vi "Averaged FFT Spectrum (Real-Im).vi"(0 "scaled signal [EU]":dbl[](array[numeric]) format="%.2f", 1 "sampling frequency [Hz]":dbl=10000.0 format="%.2f", 2 "window":T6 items=["Rectangle"=0, "Hanning"=1, "Hamming"=2, "Blackman-Harris"=3, "Exact Blackman"=4, "Blackman"=5, "Flat Top"=6, "4 Term B-Harris "=7, "7 Term B-Harris"=8, "Low Sidelobe"=9, "Blackman Nuttall"=11, "Triangle"=30, "Bartlett-Hanning"=31, "Bohman"=32, "Parzen"=33, "Welch"=34, "Kaiser"=60, "Dolph-Chebyshev"=61, "Gaussian"=62], 5 "channel info":T1={"sensor sensitivity [mV/EU]"=1000.0, "engineering units"=1, "dB reference [EU]"=1.0, "custom label"="EU", "weighting filter"=0, "pregain [dB]"=0.0} {"pregain [dB]" format="%.2f"; "weighting filter" items=["Linear", "A-weighting", "B-weighting", "C-weighting", "ITU-R 468-4", "Dolby", "CCITT", "C-message"]; "dB reference [EU]" format="%^.1e"; "engineering units" items=["custom..."=0, "V"=1, "A"=21, "Pa"=2, "N"=20, "g"=3, "m/s^2"=4, "m/s"=5, "m"=6, "mm/s"=12, "mm"=13, "microns/s"=14, "microns"=15, "in/s^2"=7, "in/s"=8, "in"=9, "mils/s"=10, "mils"=11, "rad/s^2"=16, "rad/s"=17, "rad"=18, "strain"=19]; "sensor sensitivity [mV/EU]" format="%.2f"}, 6 "frequency weighting":T5(ring), 7 "reset averaging (T)":bool=TRUE, 9 "averaging parameters":T4={"averaging mode"=enum."RMS averaging", "weighting mode"=enum."Linear", "number of averages"=10} {"number of averages" min=1}) -> (11 "window constants":cluster{"eq noise BW":dbl, "coherent gain":dbl} {"coherent gain" format="%.2f"; "eq noise BW" format="%.2f"}, 12 "df [Hz]":dbl format="%.2f", 13 "weighting conflict":bool, 14 "real part [EUrms]":dbl[](array[numeric]) format="%.2f", 15 "imaginary part [EUrms]":dbl[](array[numeric]) format="%.2f", 16 "unit label":string, 18 "averages completed":dbl format="%.2f", 19 "error out":errorcluster)   [LabVIEW 2017]
doc: "Computes the averaged FFT spectrum of the input signal. FFT results are returned as real and imaginary parts.\nEach block of data corresponds to a single FFT block and has to be passed individually to this VI. The first time this VI is called, reset averaging must be TRUE (default value), to start a new averaging process. For subsequent calls, reset averaging must be FALSE to continue the averaging process. Averages completed returns the number of averages completed so far.\nAveraging parameters specifies how the averaging is performed. This includes the averaging mode (no averaging, vector averaging, RMS averaging, or peak hold), the weighting mode (linear or exponential), and the number of averages (used only if the weighting mode is exponential).\nThe selected frequency weighting (A, B, or C) is applied to the results in the frequency domain. There is no time-domain filtering operation."
uses:
  <vilib>/Analysis/4window.llb/windowTd.ctl
  <vilib>/addons/Sound and Vibration/compatibility/Controls/svl_Channel Info.ctl
  <vilib>/addons/Sound and Vibration/compatibility/Controls/svl_Engineering Units Text Ring.ctl
  <vilib>/addons/Sound and Vibration/compatibility/Controls/svl_Weighting Filter Text Ring.ctl
  <vilib>/Analysis/2dsp.llb/Real FFT.vi
  <vilib>/Analysis/2dsp.llb/Power Spectrum (DBL).vi
  <vilib>/Analysis/0measdsp.llb/Scaled Time Domain Window (DBL).vi
  <vilib>/Analysis/NI_AALPro.lvlib
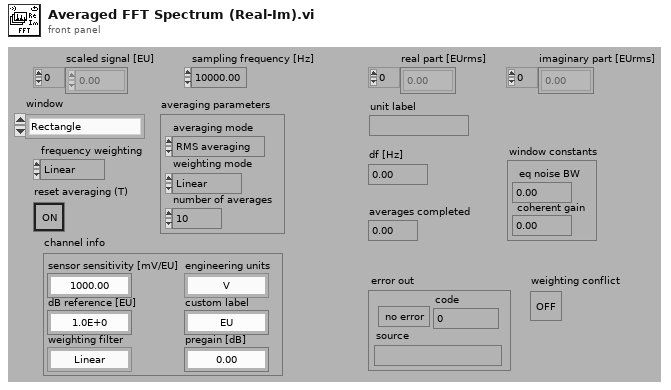
[diagram p1: front panel]
types:
  T1 = typedef "svl_Channel Info.ctl" = cluster{"sensor sensitivity [mV/EU]":dbl, "engineering units":T2, "dB reference [EU]":dbl, "custom label":string, "weighting filter":T3, "pregain [dB]":dbl}
  T2 = typedef "svl_Engineering Units Text Ring.ctl" = u16
  T3 = typedef "svl_Weighting Filter Text Ring.ctl" = u16
  T4 = cluster{"averaging mode":enum16{"No averaging", "Vector averaging", "RMS averaging", "Peak hold"}, "weighting mode":enum16{"Linear", "Exponential"}, "number of averages":u32}
  T5 = enum16{"Linear", "A-weighting", "B-weighting", "C-weighting"}
  T6 = typedef "NI_AALPro.lvlib/windowTd.ctl" = u32
  T7 = enum16{"No averaging", "Vector averaging", "RMS averaging", "Peak hold"}
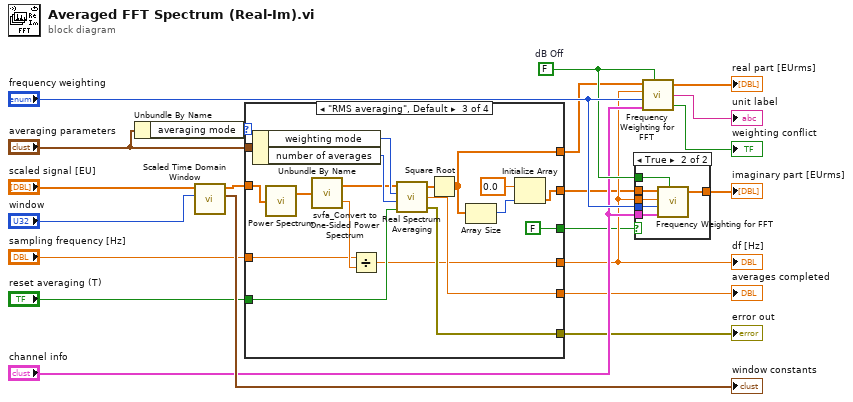
[diagram p0: block diagram]
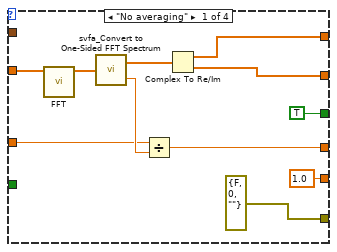
[diagram p2: hidden frame]
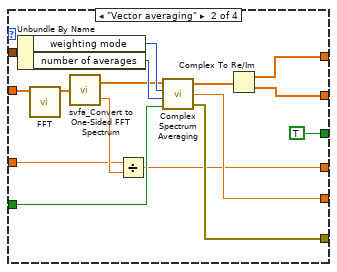
[diagram p3: hidden frame]
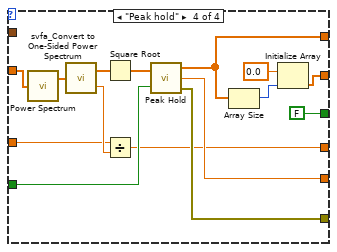
[diagram p4: hidden frame]
diagram:
  w17 = FALSE  # dB Off
  n1 = Unbundle By Name("averaging parameters") -> ("averaging mode"=w8:T7)
  n2 = call-poly <vilib>:"Scaled Time Domain Window.vi"("window"="window", "X"="scaled signal [EU]") -> ("window properties"=→"window constants":cluster{"eq noise BW":dbl, "coherent gain":dbl}, "Windowed X"=w10:dbl[])  [unwired: 7 in, 1 out]
  n3 = case shown="\"RMS averaging\", Default" w8 {
    tunnel: "sampling frequency [Hz]" -> [w23 w34 w50 w69]
    tunnel: [w22 w33 w49 w68] -> w6
    tunnel: [1.0 ("averages completed") w48 w65 w79] -> w7
    tunnel: "reset averaging (T)" -> [_ w47 w66 w80]
    tunnel: w10 -> [w25 w36 w52 w70]
    tunnel: "averaging parameters" -> [_ w46 w64 _]
    tunnel: [w31 w44 w56 w75] -> w3
    tunnel: [w30 w43 w63 w76] -> w4
    tunnel: [TRUE TRUE FALSE FALSE] -> w5
    tunnel: [errorcluster {"status"=FALSE, "code"=0, "source"=""} ("error out") w39 w59 w73] -> w2
    frame "No averaging" {
      n4 = call-poly <vilib>:"FFT.vi"("X"=w25) -> ("FFT {X}"=w27:cdb[])  [unwired: 9 in, 1 out]
      n5 = call <vilib>:"svfa_Convert to One-Sided FFT Spectrum.vi"("two-sided FFT spectrum"=w27) -> ("one-sided FFT spectrum"=w24:cdb[], "block size"=w26:dbl)
      n6 = Divide(x=w23, y=w26) -> (x/y=w22:dbl)
      n7 = Complex To Re/Im(x + iy=w24) -> (x=w31:dbl[], y=w30:dbl[])
    }
    frame "Vector averaging" {
      n8 = Unbundle By Name(w46) -> ("weighting mode"=w41:enum16{"Linear", "Exponential"}, "number of averages"=w40:u32)
      n9 = call-poly <vilib>:"FFT.vi"("X"=w36) -> ("FFT {X}"=w38:cdb[])  [unwired: 9 in, 1 out]
      n10 = call <vilib>:"svfa_Convert to One-Sided FFT Spectrum.vi"("two-sided FFT spectrum"=w38) -> ("one-sided FFT spectrum"=w35:cdb[], "block size"=w37:dbl)
      n11 = Divide(x=w34, y=w37) -> (x/y=w33:dbl)
      n12 = call <vilib>:"Complex Spectrum Averaging.vi"("reset averaging (T)"=w47, "number of averages"=w40, "weighting mode"=w41, "complex spectrum"=w35) -> ("error out"=w39:errorcluster, "averages completed"=w48:dbl, "averaged complex spectrum"=w45:cdb[])
      n13 = Complex To Re/Im(x + iy=w45) -> (x=w44:dbl[], y=w43:dbl[])
    }
    frame "RMS averaging", Default {
      n14 = Unbundle By Name(w64) -> ("weighting mode"=w55:enum16{"Linear", "Exponential"}, "number of averages"=w58:u32)
      n15 = call-poly <vilib>:"Power Spectrum.vi"("X"=w52) -> ("Power Spectrum"=w54:dbl[])  [unwired: 1 out]
      n16 = call <vilib>:"svfa_Convert to One-Sided Power Spectrum.vi"("two-sided power spectrum"=w54) -> ("one-sided power spectrum"=w51:dbl[], "block size"=w53:dbl)
      n17 = Divide(x=w50, y=w53) -> (x/y=w49:dbl)
      n18 = call <vilib>:"Real Spectrum Averaging.vi"("reset averaging (T)"=w66, "number of averages"=w58, "weighting mode"=w55, "real spectrum"=w51) -> ("error out"=w59:errorcluster, "averages completed"=w65:dbl, "averaged real spectrum"=w57:dbl[])
      n19 = Square Root(x=w57) -> (sqrt(x)=w56:dbl[])
      n20 = Array Size(array=w56) -> (size(s)=w61:i32)
      n21 = Initialize Array(0.0, w61) -> (w63:dbl[])
    }
    frame "Peak hold" {
      n22 = call-poly <vilib>:"Power Spectrum.vi"("X"=w70) -> ("Power Spectrum"=w72:dbl[])  [unwired: 1 out]
      n23 = call <vilib>:"svfa_Convert to One-Sided Power Spectrum.vi"("two-sided power spectrum"=w72) -> ("one-sided power spectrum"=w67:dbl[], "block size"=w71:dbl)
      n24 = Square Root(x=w67) -> (sqrt(x)=w81:dbl[])
      n25 = Divide(x=w69, y=w71) -> (x/y=w68:dbl)
      n26 = call <vilib>:"Peak Hold.vi"("real spectrum"=w81, "reset averaging"=w80) -> ("peak spectrum"=w75:dbl[], "averages completed"=w79:dbl, "error out"=w73:errorcluster)
      n27 = Array Size(array=w75) -> (size(s)=w77:i32)
      n28 = Initialize Array(0.0, w77) -> (w76:dbl[])
    }
  }
  "df [Hz]" <- w6
  "averages completed" <- w7
  "error out" <- w2
  n29 = case shown="True" w5 {
    tunnel: "channel info" -> [_ w88]
    tunnel: [w82 w87] -> w19
    tunnel: "frequency weighting" -> [_ w86]
    tunnel: w17 -> [_ w85]
    tunnel: w6 -> [_ w84]
    tunnel: w4 -> [w82 w83]
    frame False {
    }
    frame True {
      n30 = call <vilib>:"Frequency Weighting for FFT.vi"("FFT [EUrms]"=w83, "df [Hz]"=w84, "frequency weighting"=w86, "channel info"=w88, "dB On (F)"=w85) -> ("frequency weighted FFT [EUrms]"=w87:dbl[])  [unwired: 2 out]
    }
  }
  "imaginary part [EUrms]" <- w19
  n31 = call <vilib>:"Frequency Weighting for FFT.vi"("FFT [EUrms]"=w3, "df [Hz]"=w6, "frequency weighting"="frequency weighting", "channel info"="channel info", "dB On (F)"=w17) -> ("frequency weighted FFT [EUrms]"=→"real part [EUrms]":dbl[], "unit label"=→"unit label":string, "weighting conflict"=→"weighting conflict":bool)
